vi "ECOG-Restore Settings.vi"() -> (8 "Settings":T1)   [LabVIEW 2020]
uses:
  Typedefs/ECOG-Parameters.ctl
panel:
  in  "Defaults":T1={"Channel"="", "Fs"=1000.0, "Frame Size"=100.0, "History Length"=5.0, "Filter"=TRUE, "Flo"=0.1, "Fhi"=30.0, "Fmax"=0.0, "Splitter Position"=0}
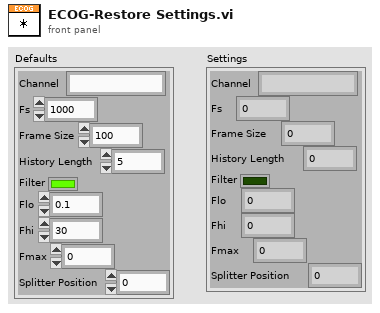
[diagram p1: front panel]
types:
  T1 = typedef "ECOG-Parameters.ctl" = cluster{"Channel":string, "Fs":dbl, "Frame Size":dbl, "History Length":dbl, "Filter":bool, "Flo":dbl, "Fhi":dbl, "Fmax":dbl, "Splitter Position":i32}
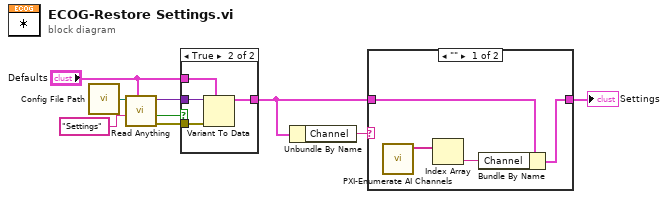
[diagram p0: block diagram]
diagram:
  n1 = call "Config File Path.vi"() -> ("Default config file name"=w4:path)  [unwired: 1 in]
  n2 = call "Read Anything.vi"("Type of Anything"="Defaults", "Section Name (Name of \"Type of Anything\")"="Settings" ("Section Name (Name of \"Type of Anything\")"), "Path (dialog)"=w4) -> ("Error Out"=w9:errorcluster, "Found?"=w8:bool, "Anything"=w6:variant)  [unwired: 6 in]
  n3 = case shown="True" w8 {
    tunnel: w6 -> [_ w13]
    tunnel: "Defaults" -> [w10 w12]
    tunnel: w9 -> [_ w14]
    tunnel: [w10 w11] -> w2
    frame False {
    }
    frame True {
      n4 = Variant To Data(error in=w14, type=w12, Variant=w13) -> (data=w11:T1)  [unwired: 1 out]
    }
  }
  n5 = Unbundle By Name(w2) -> ("Channel"=w3:string)
  n6 = case shown="\"\"" w3 {
    tunnel: w2 -> [w18 w19]
    tunnel: [w17 w19] -> w1
    frame "" {
      n7 = call "PXI-Enumerate AI Channels.vi"() -> ("AI.PhysicalChans"=w16:tag[])  [unwired: 11 in]
      n8 = Index Array(array=w16) -> (element=w15:tag)  [unwired: 1 in]
      n9 = Bundle By Name(cluster=w18, "Channel"=w15) -> (w17:T1)
    }
    frame Default {
    }
  }
  "Settings" <- w1
